vi "P10 Global 1.vi"() -> ()   [LabVIEW 2019]
panel:
  in  "Position":dbl
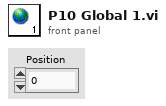
[diagram p1: front panel]
diagram:
